vi "Log Result.vi"(8 "error in (no error)":errorcluster, 10 "tdms file":refnum<k34>, 11 "Waveform Array Result in":refnum<class "Waveform Array Result.lvclass">) -> (0 "error out":errorcluster, 2 "tdms file out":refnum<k34>, 3 "Waveform Array Result out":refnum<class "Waveform Array Result.lvclass">)   [LabVIEW 2015, in "Waveform Array Result.lvclass"]
uses:
  Waveform Array Result.lvclass
  Mag Lab Result.lvclass/Mag Lab Result.ctl
  Waveform Array Result.lvclass/Waveform Array Result.ctl
  Read Group Name.vi
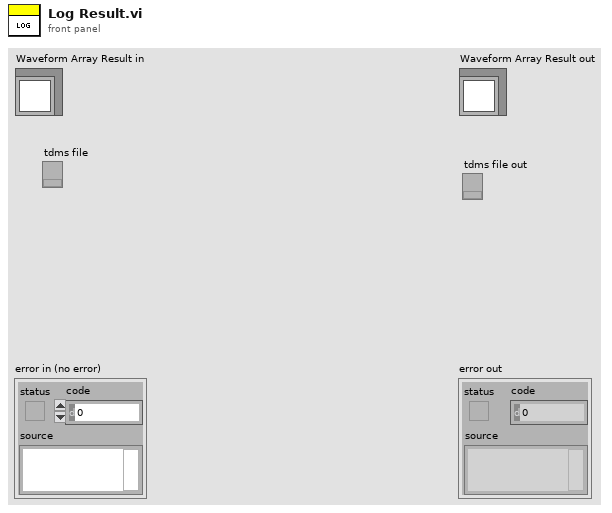
[diagram p1: front panel]
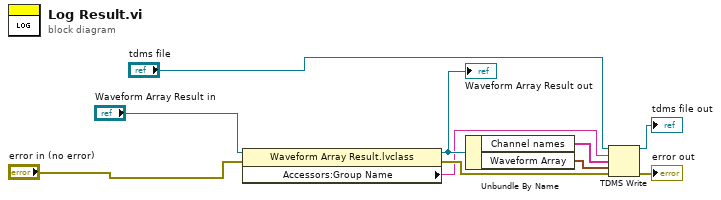
[diagram p0: block diagram]
diagram:
  n1 = property class="Waveform Array Result.lvclass"(reference="Waveform Array Result in", error in="error in (no error)") -> (reference out=w6:refnum<class "Waveform Array Result.lvclass">, error out=w5:errorcluster, "Accessors:Group Name"=w4:string)
  "Waveform Array Result out" <- w6
  n2 = Unbundle By Name(w6) -> ("Channel names"=w9:string[], "Waveform Array"=w8:waveform(dbl)[])
  n3 = TDMS Write(0:"tdms file", 5:w4, 7:w9, 9:w8, 11:w5) -> (4:→"tdms file out":refnum<k34>, 15:→"error out":errorcluster)  [unwired: 1 in, 2 out]
